vi "Scan Housing Type.vi"(10 "Lookup Path In":path) -> (0 "OK?":bool, 2 "Housing Type Out":string)   [LabVIEW 2024, in "LVarex.lvlib"]
uses:
  LVarex.lvlib
panel:
  out "First Scan?":bool
  in  "Case Constant\n(See Context Help)":bool
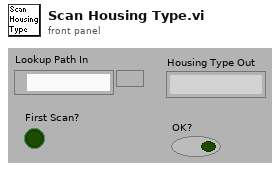
[diagram p1: front panel]
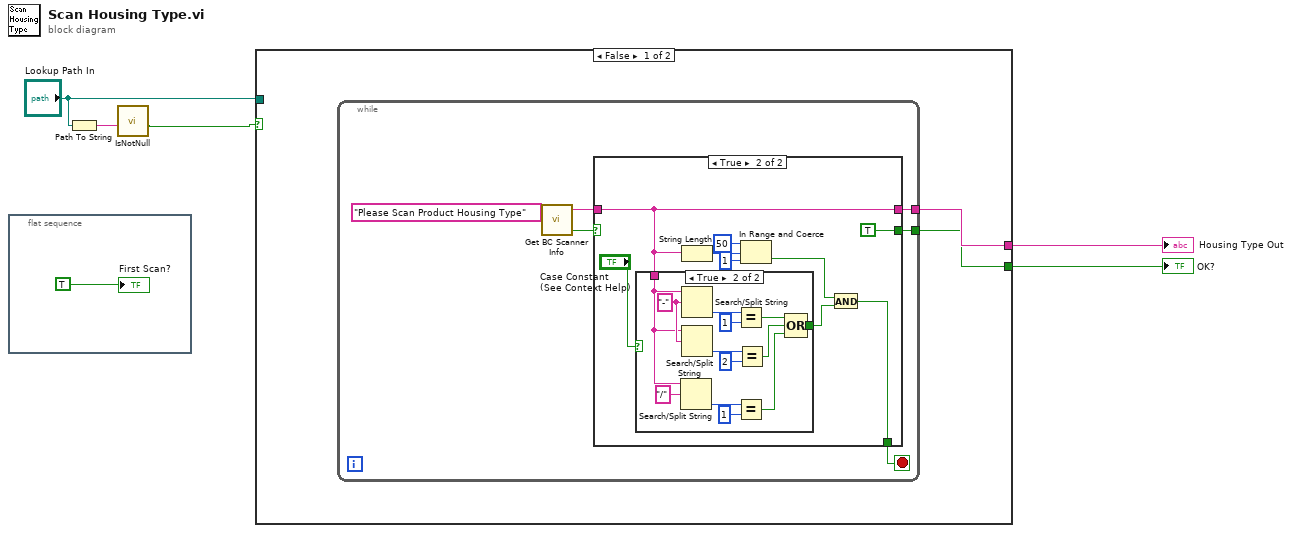
[diagram p0: block diagram]
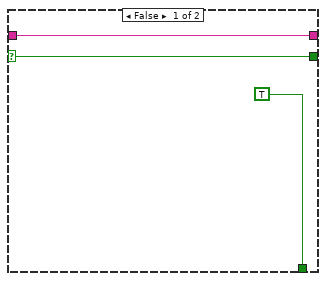
[diagram p2: hidden frame]
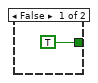
[diagram p3: hidden frame]
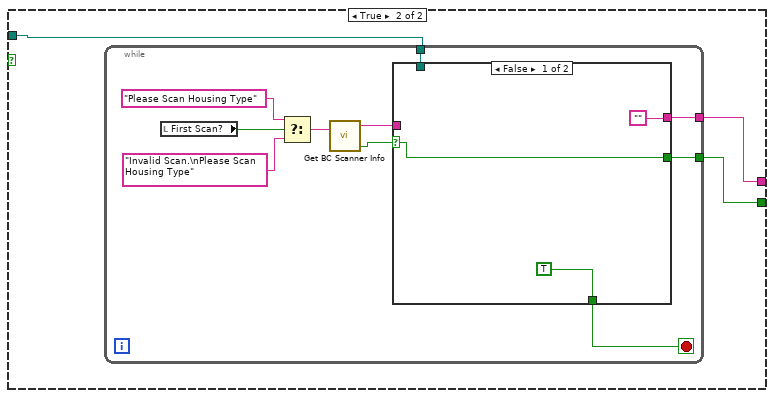
[diagram p4: hidden frame]
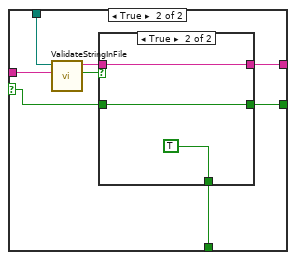
[diagram p5: hidden frame]
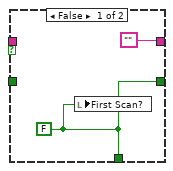
[diagram p6: hidden frame]
diagram:
  n1 = flat-sequence {
    frame #0 {
      "First Scan?" <- TRUE
    }
  }
  n2 = Path To String(path="Lookup Path In") -> (string=w2:string)
  n3 = call "IsNotNull.vi"("String In"=w2) -> ("Boolean Out"=w1:bool)  [unwired: 10 in]
  n4 = case shown="False" w1 {
    tunnel: [w8 w42] -> w5
    tunnel: [w7 w41] -> w4
    tunnel: "Lookup Path In" -> [_ w43]
    frame False {
      n5 = while {
        tunnel: [w11] -> w7
        tunnel: [w10] -> w8
        stop <- w9 stop-if-true
        n6 = call "Get BC Scanner Info.vi"("Prompt"="Please Scan Product Housing Type") -> ("Info Out"=w12:string, "OK"=w13:bool)  [unwired: 2 in]
        n7 = case shown="True" w13 {
          selector: w13 -> [w17 _]
          tunnel: w12 -> [w16 w20]
          tunnel: [w17 TRUE] -> w11
          tunnel: [w16 w20] -> w10
          tunnel: [TRUE w21] -> w9
          frame False {
          }
          frame True {
            n8 = case shown="True" "Case Constant\n(See Context Help)" {
              tunnel: w20 -> [_ w33]
              tunnel: [TRUE w28] -> w19
              frame False {
              }
              frame True {
                w40 = "-" ("search string/char (-)")
                n9 = Search/Split String(string=w33, search string/char (-)="/") -> (offset of match=w34:i32)  [unwired: 1 in, 2 out]
                n10 = Search/Split String(string=w33, search string/char (-)=w40) -> (offset of match=w39:i32)  [unwired: 1 in, 2 out]
                n11 = Search/Split String(string=w33, search string/char (-)=w40) -> (offset of match=w38:i32)  [unwired: 1 in, 2 out]
                n12 = Equal?(x=w39, y=1) -> (x = y?=w31:bool)
                n13 = Equal?(x=w34, y=1) -> (x = y?=w29:bool)
                n14 = Equal?(x=w38, y=2) -> (x = y?=w30:bool)
                n15 = Compound Arithmetic op=OR(w31, w30, w29) -> (w28:bool)
              }
            }
            n16 = String Length(string=w20) -> (length=w25:i32)
            n17 = In Range and Coerce(upper limit=50, x=w25, lower limit=1) -> (In Range?=w22:bool)  [unwired: 1 out]
            n18 = And(x=w22, y=w19) -> (x .and. y?=w21:bool)
          }
        }
      }
    }
    frame True {
      n19 = while {
        tunnel: w43 -> [w47]
        tunnel: [w46] -> w42
        tunnel: [w45] -> w41
        stop <- w44 stop-if-true
        n20 = local read "First Scan?"() -> (w52:bool)
        n21 = Select(t="Please Scan Housing Type", s=w52, f="Invalid Scan.\nPlease Scan Housing Type") -> (s? t:f=w50:string)
        n22 = call "Get BC Scanner Info.vi"("Prompt"=w50) -> ("Info Out"=w48:string, "OK"=w49:bool)  [unwired: 2 in]
        n23 = case shown="False" w49 {
          selector: w49 -> [w55 w59]
          tunnel: w48 -> [_ w64]
          tunnel: w47 -> [_ w63]
          tunnel: ["" w60] -> w46
          tunnel: [w55 w58] -> w45
          tunnel: [TRUE w57] -> w44
          frame False {
          }
          frame True {
            n24 = call "ValidateStringInFile.vi"("String to find"=w64, "Path In"=w63) -> ("String Found"=w62:bool, "String Out"=w61:string)  [unwired: 7 in, 1 out]
            n25 = case shown="True" w62 {
              tunnel: w61 -> [_ w69]
              tunnel: ["" w69] -> w60
              tunnel: w59 -> [_ w68]
              tunnel: [w65 w68] -> w58
              tunnel: [w65 TRUE] -> w57
              frame False {
                w65 = FALSE
                n26 = local write "First Scan?"(w65) -> ()
              }
              frame True {
              }
            }
          }
        }
      }
    }
  }
  "Housing Type Out" <- w5
  "OK?" <- w4
